vi "Get Database Manager.vi"(8 "error in (no error)":errorcluster, 11 "Attributes in":refnum<class "Attributes.lvclass">) -> (0 "error out":errorcluster, 2 "Database Manager":refnum<class "Database Manager.lvclass">, 3 "Attributes out":refnum<class "Attributes.lvclass">)   [LabVIEW 2019, in "HierDAL Library.lvlib" / "Database.lvlib" / "Repositories.lvlib" / "Attributes.lvclass"]
uses:
  Attributes.lvclass
  Database Manager Class/Database Manager.lvclass
  Attributes.lvclass/Attributes.ctl
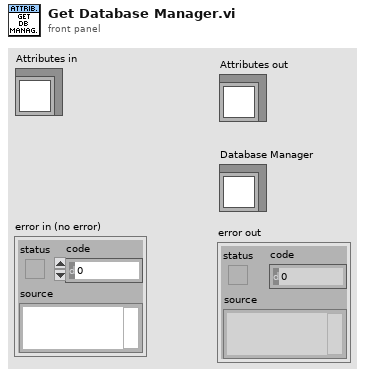
[diagram p1: front panel]
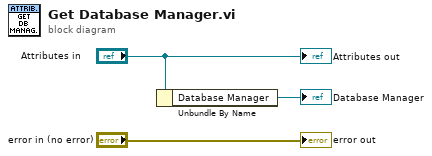
[diagram p0: block diagram]
diagram:
  n1 = Unbundle By Name("Attributes in") -> ("Database Manager"=→"Database Manager":refnum<class "Database Manager.lvclass">)
  "error out" <- "error in (no error)"
  "Attributes out" <- "Attributes in"
